vi "RTSPInterface.vi"() -> ()   [LabVIEW 2010]
panel:
  in  "Stop receiving":bool
  in  "millisecond delay":u32
  out "millisecond timer value":u32
  in  "?":bool
  in  "?":bool
  out "Message  sent":string
  out "Unknown Message Received":string
  in  "RemotePort":u16=50010
  in  "Local Sending Port":u16=49999
  out "loops/ms":dbl
  out "error out":errorcluster
  out "Received Message":string
  in  "max bytes/read":i32=548
  out "# of Bytes Received":i32
  in  "Local Receiving Port":u16=50011
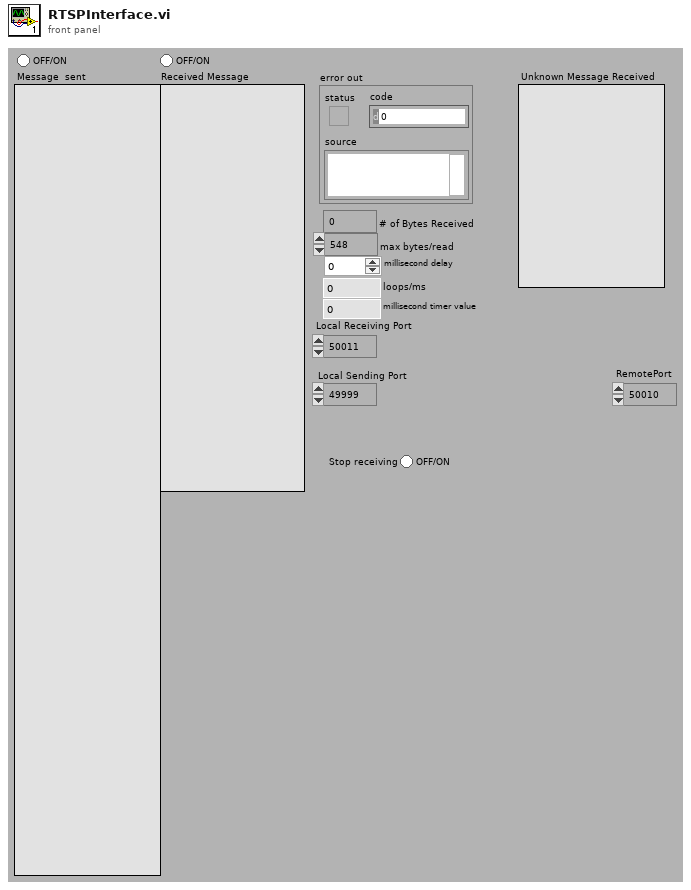
[diagram p1: front panel]
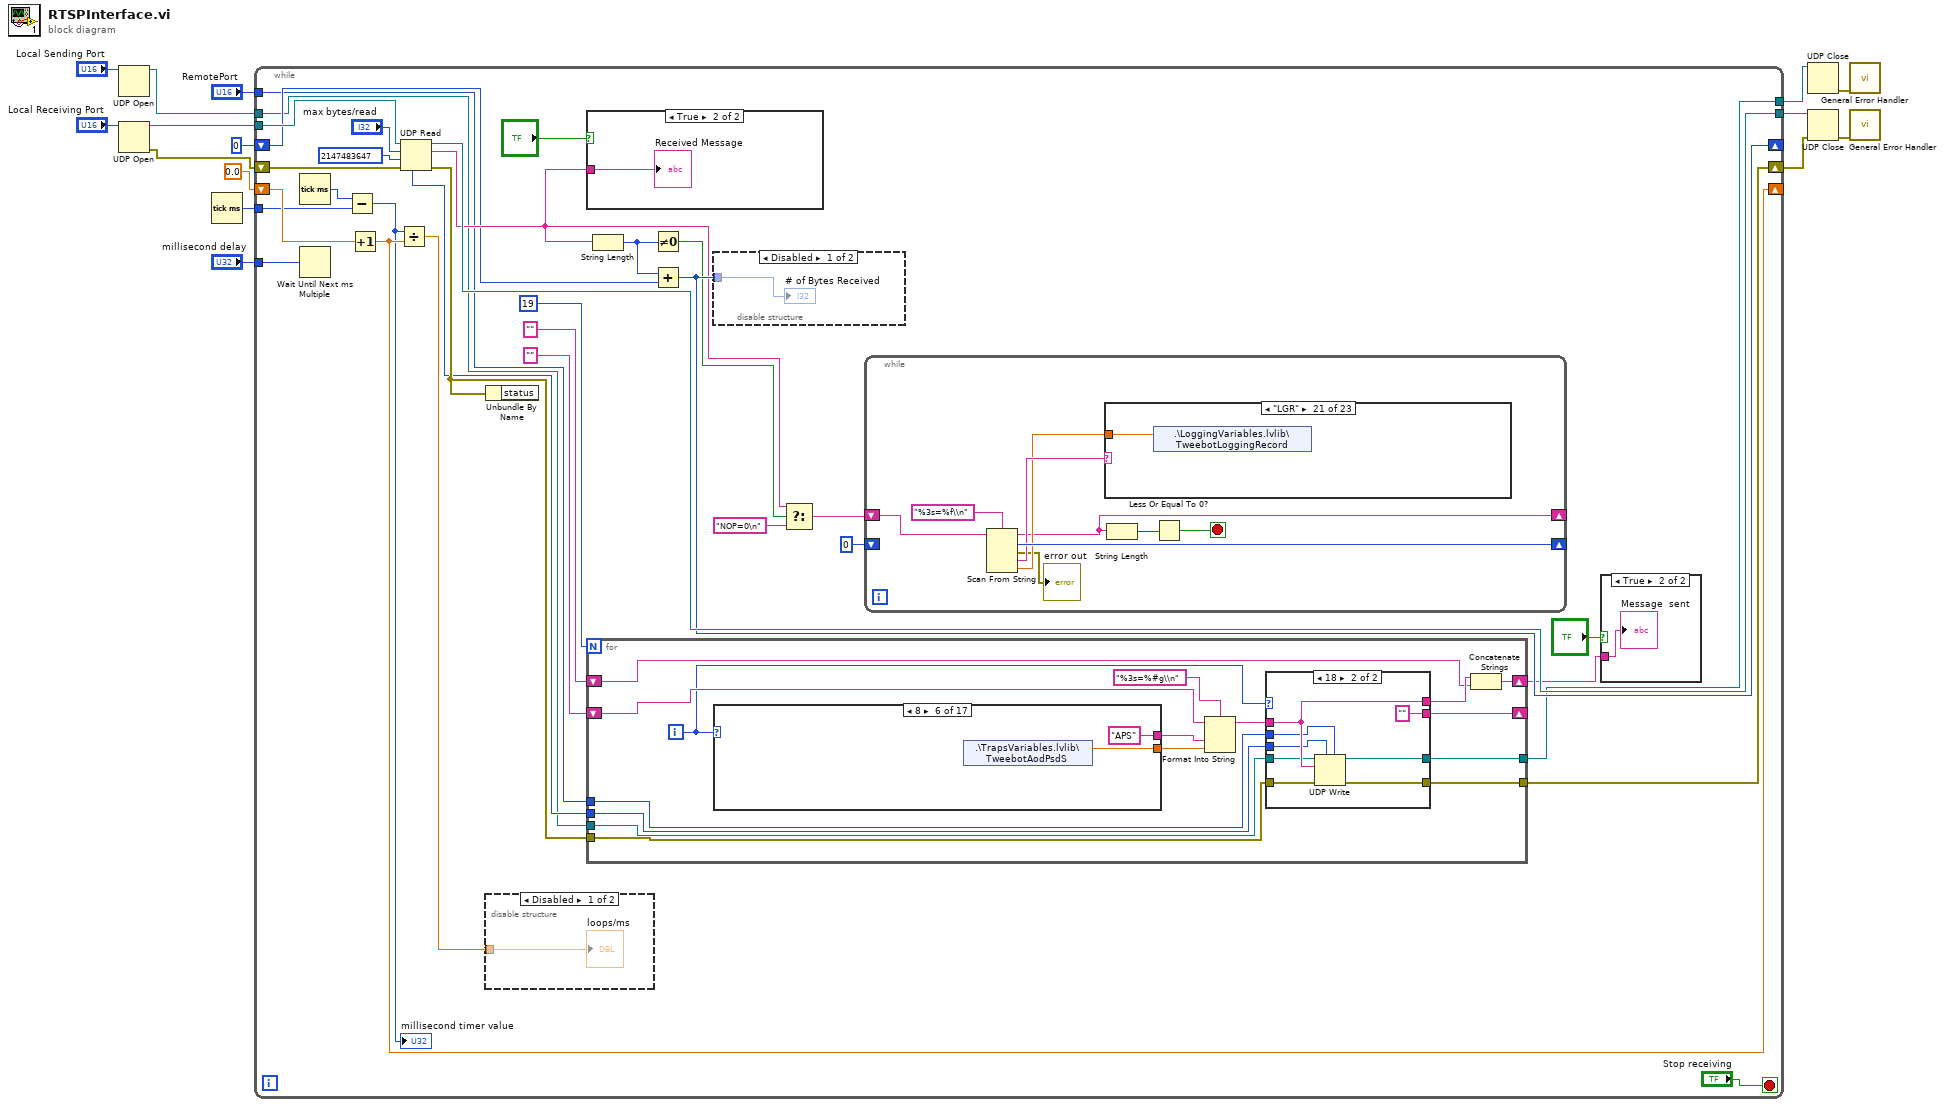
[diagram p0: block diagram]
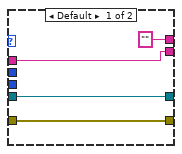
[diagram p5: hidden frame]
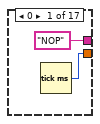
[diagram p6: hidden frame]
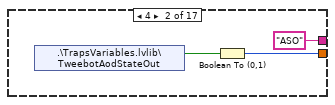
[diagram p7: hidden frame]
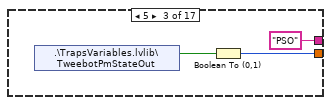
[diagram p8: hidden frame]
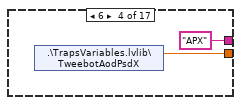
[diagram p9: hidden frame]
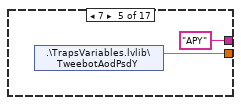
[diagram p10: hidden frame]
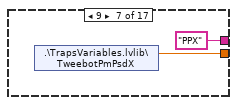
[diagram p11: hidden frame]
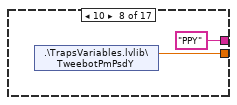
[diagram p12: hidden frame]
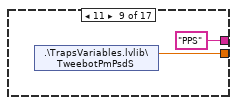
[diagram p13: hidden frame]
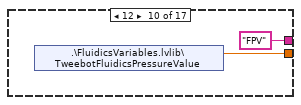
[diagram p14: hidden frame]
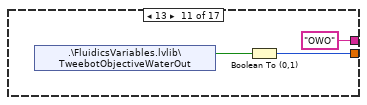
[diagram p15: hidden frame]
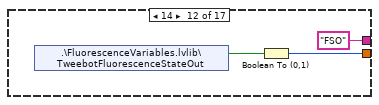
[diagram p16: hidden frame]
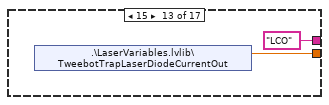
[diagram p17: hidden frame]
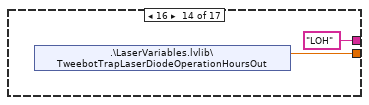
[diagram p18: hidden frame]
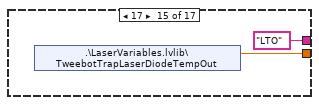
[diagram p19: hidden frame]
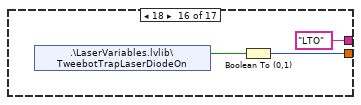
[diagram p20: hidden frame]
diagram:
  n1 = UDP Open(11:"Local Sending Port") -> (port=w2:refnum<k16>)  [unwired: 1 in, 5 out]
  n2 = UDP Open(11:"Local Receiving Port") -> (port=w14:refnum<k16>, 0:w15:errorcluster)  [unwired: 4 in, 1 out]
  n3 = Tick Count (ms)() -> (millisecond timer value=w5:u32)
  n4 = while {
    shift-left: 0 -> [w33]
    shift-right: [w43] -> _
    tunnel: [w46] -> w13
    tunnel: w14 -> [w47]
    shift-left: w15 -> [w48]
    shift-right: [w21] -> w12
    shift-right: [w35] -> _
    shift-left: 0.0 -> [w36]
    tunnel: w5 -> [w30]
    tunnel: "millisecond delay" -> [w28]
    tunnel: "RemotePort" -> [w18]
    tunnel: w2 -> [w17]
    tunnel: [w16] -> w1
    stop <- "Stop receiving" stop-if-true
    n5 = Tick Count (ms)() -> (millisecond timer value=w29:u32)
    n6 = Wait Until Next ms Multiple(millisecond multiple=w28) -> ()  [unwired: 1 out]
    n7 = Subtract(x=w29, y=w30) -> (x-y=w31:u32)
    "millisecond timer value" <- w31
    n8 = Increment(x=w36) -> (x+1=w35:dbl)
    n9 = Divide(x=w31, y=w35) -> (x/y=w34:dbl)
    n10 = UDP Read(connection ID=w47, max size (548)="max bytes/read", timeout ms (25000)=2147483647, 8:w48) -> (data out=w40:string, error out=w20:errorcluster, 3:w46:refnum<k16>, 6:w19:u32)  [unwired: 1 out]
    n11 = Unbundle By Name(w20) -> ()  [unwired: 1 out]
    n12 = disable-structure shown="Disabled" {
      disable-tunnel: w34 -> [w50 _]
      frame Disabled {
        "loops/ms" <- w50
      }
      frame Enabled {
      }
    }
    n13 = case shown="True" "?" {
      tunnel: w40 -> [_ w119]
      frame False {
      }
      frame True {
        "Received Message" <- w119
      }
    }
    n14 = for {
      N: 19 -> [_]
      shift-right: [w58] -> _
      shift-left: "" -> [w67]
      tunnel: w20 -> [w62]
      tunnel: [w61] -> w16
      tunnel: [w60] -> w21
      shift-right: [w55] -> w24
      shift-left: "" -> [w56]
      tunnel: w19 -> [w54]
      tunnel: w18 -> [w53]
      tunnel: w17 -> [w52]
      i -> [w63]
      n15 = case shown="8" w63 {
        tunnel: [w80 w82 w85 w89 w91 w93 w95 w97 w99 w100 w102 w105 w108 w110 w112 w114 w117] -> w66
        tunnel: ["NOP" ("format string") "ASO" ("format string") "PSO" ("format string") "APX" ("format string") "APY" ("format string") "APS" ("format string") "PPX" ("format string") "PPY" ("format string") "PPS" ("format string") "FPV" ("format string") "OWO" ("format string") "FSO" ("format string") "LCO" ("format string") "LOH" ("format string") "LTO" ("format string") "LTO" ("format string") "NOP" ("format string")] -> w65
        frame 0 {
          n16 = Tick Count (ms)() -> (millisecond timer value=w80:u32)
        }
        frame 4 {
          n17 = shared-variable ".\\TrapsVariables.lvlib\\TweebotAodStateOut"() -> (w83:bool)  [unwired: 1 in, 1 out]
          n18 = Boolean To (0,1)(Boolean=w83) -> (0, 1=w82:i16)
        }
        frame 5 {
          n19 = shared-variable ".\\TrapsVariables.lvlib\\TweebotPmStateOut"() -> (w86:bool)  [unwired: 1 in, 1 out]
          n20 = Boolean To (0,1)(Boolean=w86) -> (0, 1=w85:i16)
        }
        frame 6 {
          n21 = shared-variable ".\\TrapsVariables.lvlib\\TweebotAodPsdX"() -> (w89:dbl)  [unwired: 1 in, 1 out]
        }
        frame 7 {
          n22 = shared-variable ".\\TrapsVariables.lvlib\\TweebotAodPsdY"() -> (w91:dbl)  [unwired: 1 in, 1 out]
        }
        frame 8 {
          n23 = shared-variable ".\\TrapsVariables.lvlib\\TweebotAodPsdS"() -> (w93:dbl)  [unwired: 1 in, 1 out]
        }
        frame 9 {
          n24 = shared-variable ".\\TrapsVariables.lvlib\\TweebotPmPsdX"() -> (w95:dbl)  [unwired: 1 in, 1 out]
        }
        frame 10 {
          n25 = shared-variable ".\\TrapsVariables.lvlib\\TweebotPmPsdY"() -> (w97:dbl)  [unwired: 1 in, 1 out]
        }
        frame 11 {
          n26 = shared-variable ".\\TrapsVariables.lvlib\\TweebotPmPsdS"() -> (w99:dbl)  [unwired: 1 in, 1 out]
        }
        frame 12 {
          n27 = shared-variable ".\\FluidicsVariables.lvlib\\TweebotFluidicsPressureValue"() -> (w100:dbl)  [unwired: 1 in, 1 out]
        }
        frame 13 {
          n28 = shared-variable ".\\FluidicsVariables.lvlib\\TweebotObjectiveWaterOut"() -> (w103:bool)  [unwired: 1 in, 1 out]
          n29 = Boolean To (0,1)(Boolean=w103) -> (0, 1=w102:i16)
        }
        frame 14 {
          n30 = shared-variable ".\\FluorescenceVariables.lvlib\\TweebotFluorescenceStateOut"() -> (w106:bool)  [unwired: 1 in, 1 out]
          n31 = Boolean To (0,1)(Boolean=w106) -> (0, 1=w105:i16)
        }
        frame 15 {
          n32 = shared-variable ".\\LaserVariables.lvlib\\TweebotTrapLaserDiodeCurrentOut"() -> (w108:dbl)  [unwired: 1 in, 1 out]
        }
        frame 16 {
          n33 = shared-variable ".\\LaserVariables.lvlib\\TweebotTrapLaserDiodeOperationHoursOut"() -> (w110:dbl)  [unwired: 1 in, 1 out]
        }
        frame 17 {
          n34 = shared-variable ".\\LaserVariables.lvlib\\TweebotTrapLaserDiodeTempOut"() -> (w112:dbl)  [unwired: 1 in, 1 out]
        }
        frame 18 {
          n35 = shared-variable ".\\LaserVariables.lvlib\\TweebotTrapLaserDiodeOn"() -> (w115:bool)  [unwired: 1 in, 1 out]
          n36 = Boolean To (0,1)(Boolean=w115) -> (0, 1=w114:i16)
        }
        frame Default {
          n37 = Tick Count (ms)() -> (millisecond timer value=w117:u32)
        }
      }
      n38 = Format Into String(format string="%3s=%#g\\n", initial string=w67, w65, w66) -> (resulting string=w59:string)  [unwired: 1 in, 1 out]
      n39 = case shown="18" w63 {
        tunnel: w62 -> [w70 w79]
        tunnel: w59 -> [w71 w75]
        tunnel: [w68 w78] -> w61
        tunnel: [w70 w77] -> w60
        tunnel: [w71 ""] -> w58
        tunnel: ["" w75] -> w57
        tunnel: w54 -> [_ w74]
        tunnel: w53 -> [_ w73]
        tunnel: w52 -> [w68 w72]
        frame Default {
        }
        frame 18 {
          n40 = UDP Write(address=w74, port or service name=w73, connection ID=w72, data in=w75, 8:w79) -> (error out=w77:errorcluster, 3:w78:refnum<k16>)  [unwired: 1 out]
        }
      }
      n41 = Concatenate Strings(w57, w56) -> (w55:string)
    }
    n42 = String Length(string=w40) -> (length=w37:i32)
    n43 = Not Equal To 0?(x=w37) -> (x != 0?=w41:bool)
    n44 = Add(x=w37, y=w33) -> (x+y=w43:i32)
    n45 = disable-structure shown="Disabled" {
      disable-tunnel: w43 -> [w49 _]
      frame Disabled {
        "# of Bytes Received" <- w49
      }
      frame Enabled {
      }
    }
    n46 = Select(t=w40, s=w41, f="NOP=0\n") -> (s? t:f=w38:string)
    n47 = while {
      shift-right: [w123] -> _
      shift-left: w38 -> [w120]
      shift-right: [w127] -> _
      shift-left: u32 0 -> [_]
      stop <- w122 stop-if-true
      n48 = Scan From String(format string="%3s=%f\\n", input string=w120) -> (remaining string=w123:string, offset past scan=w127:u32, error out=→"error out":errorcluster, output 1=w126:string, output 2=w125:dbl)  [unwired: 4 in]
      n49 = case shown="\"LGR\"" w126 {
        selector: w126 -> [_ _ _ _ _ _ _ _ _ _ _ _ _ _ _ _ _ _ _ _ _ _ w162]
        tunnel: w125 -> [w129 w131 w133 w135 w137 w138 w140 w142 w144 w145 w146 w147 w148 w149 w151 w153 w155 w157 w159 w160 w161 _ _]
        frame "FPT" {
          n50 = shared-variable ".\\FluidicsVariables.lvlib\\TweebotFluidicsPressureTime"(w129) -> ()  [unwired: 1 in, 1 out]
        }
        frame "OWI" {
          n51 = Greater Than 0?(x=w131) -> (x > 0?=w130:bool)
          n52 = shared-variable ".\\FluidicsVariables.lvlib\\TweebotObjectiveWaterIn"(w130) -> ()  [unwired: 1 in, 1 out]
        }
        frame "FPU" {
          n53 = Greater Than 0?(x=w133) -> (x > 0?=w132:bool)
          n54 = shared-variable ".\\FluidicsVariables.lvlib\\TweebotFluidicsPressureUp"(w132) -> ()  [unwired: 1 in, 1 out]
        }
        frame "FPD" {
          n55 = Greater Than 0?(x=w135) -> (x > 0?=w134:bool)
          n56 = shared-variable ".\\FluidicsVariables.lvlib\\TweebotFluidicsPressureDown"(w134) -> ()  [unwired: 1 in, 1 out]
        }
        frame "FPO" {
          n57 = Greater Than 0?(x=w137) -> (x > 0?=w136:bool)
          n58 = shared-variable ".\\FluidicsVariables.lvlib\\TweebotFluidicsPressureOpen"(w136) -> ()  [unwired: 1 in, 1 out]
        }
        frame "ASI" {
          n59 = Greater Than 0?(x=w138) -> (x > 0?=w139:bool)
          n60 = shared-variable ".\\TrapsVariables.lvlib\\TweebotAodStateIn"(w139) -> ()  [unwired: 1 in, 1 out]
        }
        frame "ATI" {
          n61 = shared-variable ".\\TrapsVariables.lvlib\\TweebotAodIntensity"(w140) -> ()  [unwired: 1 in, 1 out]
        }
        frame "PSI" {
          n62 = Greater Than 0?(x=w142) -> (x > 0?=w141:bool)
          n63 = shared-variable ".\\TrapsVariables.lvlib\\TweebotPmStateIn"(w141) -> ()  [unwired: 1 in, 1 out]
        }
        frame "FSI" {
          n64 = Greater Than 0?(x=w144) -> (x > 0?=w143:bool)
          n65 = shared-variable ".\\FluorescenceVariables.lvlib\\TweebotFluorescenceStateIn"(w143) -> ()  [unwired: 1 in, 1 out]
        }
        frame "ATX" {
          n66 = shared-variable ".\\TrapsVariables.lvlib\\TweebotAodTargetX"(w145) -> ()  [unwired: 1 in, 1 out]
        }
        frame "ATY" {
          n67 = shared-variable ".\\TrapsVariables.lvlib\\TweebotAodTargetY"(w146) -> ()  [unwired: 1 in, 1 out]
        }
        frame "PTX" {
          n68 = shared-variable ".\\TrapsVariables.lvlib\\TweebotPmTargetX"(w147) -> ()  [unwired: 1 in, 1 out]
        }
        frame "PTY" {
          n69 = shared-variable ".\\TrapsVariables.lvlib\\TweebotPmTargetY"(w148) -> ()  [unwired: 1 in, 1 out]
        }
        frame "LCI" {
          n70 = shared-variable ".\\LaserVariables.lvlib\\TweebotTrapLaserDiodeCurrentIn"(w149) -> ()  [unwired: 1 in, 1 out]
        }
        frame "LCS" {
          n71 = Greater Than 0?(x=w151) -> (x > 0?=w150:bool)
          n72 = shared-variable ".\\LaserVariables.lvlib\\TweebotTrapLaserDiodeSetCurrentIn"(w150) -> ()  [unwired: 1 in, 1 out]
        }
        frame "LNO" {
          n73 = Greater Than 0?(x=w153) -> (x > 0?=w152:bool)
          n74 = shared-variable ".\\LoggingVariables.lvlib\\TweebotLoggingNormalOnOff"(w152) -> ()  [unwired: 1 in, 1 out]
        }
        frame "LNF" {
          n75 = To Long Integer(number=w155) -> (32bit integer=w154:i32)
          n76 = shared-variable ".\\LoggingVariables.lvlib\\TweebotLoggingNormalFreq"(w154) -> ()  [unwired: 1 in, 1 out]
        }
        frame "LHO" {
          n77 = Greater Than 0?(x=w157) -> (x > 0?=w156:bool)
          n78 = shared-variable ".\\LoggingVariables.lvlib\\TweebotLoggingHighOnOff"(w156) -> ()  [unwired: 1 in, 1 out]
        }
        frame "LHF" {
          n79 = To Long Integer(number=w159) -> (32bit integer=w158:i32)
          n80 = shared-variable ".\\LoggingVariables.lvlib\\TweebotLoggingHighFreq"(w158) -> ()  [unwired: 1 in, 1 out]
        }
        frame "LGI" {
          n81 = shared-variable ".\\LoggingVariables.lvlib\\TweebotLoggingIndex"(w160) -> ()  [unwired: 1 in, 1 out]
        }
        frame "LGR" {
          n82 = shared-variable ".\\LoggingVariables.lvlib\\TweebotLoggingRecord"(w161) -> ()  [unwired: 1 in, 1 out]
        }
        frame "NOP" {
        }
        frame Default {
          "Unknown Message Received" <- w162
        }
      }
      n83 = String Length(string=w123) -> (length=w124:i32)
      n84 = Less Or Equal To 0?(x=w124) -> (x <= 0?=w122:bool)
    }
    n85 = case shown="True" "?" {
      tunnel: w24 -> [_ w51]
      frame False {
      }
      frame True {
        "Message  sent" <- w51
      }
    }
  }
  n86 = UDP Close(connection ID=w1) -> (error out=w9:errorcluster)  [unwired: 1 in, 1 out]
  n87 = UDP Close(connection ID=w13, 8:w12) -> (error out=w11:errorcluster)  [unwired: 1 out]
  n88 = call <vilib>:"General Error Handler.vi"("error in (no error)"=w9) -> ()  [unwired: 1 in, 14 out]
  n89 = call <vilib>:"General Error Handler.vi"("error in (no error)"=w11) -> ()  [unwired: 10 in, 5 out]
